vi "Main.vi"() -> ()   [LabVIEW 2020, in "ZLG_CAN.lvlib"]
doc: "This template is based off of the Queued Message Handler design pattern and the Queued Message Handler project template that ships with LabVIEW.\n\nThe main difference is that the queue is private to this module and communication between modules is performed via Broadcast and Request events.\n\nRequest events are wrapped in public API methods and are handled in the Event Handling Loop (EHL) of this VI. Any module can register for Broadcast events sent by this module. The EHL generates messages based on user interface actions.\n\nThe Message Handling Loop (MHL) processes messages generated by the EHL, or by other messages. The messages are string values, so new messages can be added easily to the Message Cases case structure in the MHL. Each message cluster can also provide an optional value for Message Data, which is a variant that can be converted to whatever message-specific data is required.\n_____\nBased on Delacor QMH Project Template 4.1.0.59."
uses:
  ZLG_CAN.lvlib
  <vilib>/Delacor/Delacor QMH/Libraries/Module Admin_class/Delacor_lib_QMH_Module Admin.lvclass
  CAN_OBJ_R.ctl
  Module Data--cluster.ctl
  <vilib>/Delacor/Delacor QMH/Libraries/Message Queue_class/Delacor_lib_QMH_Message Queue.lvclass/Delacor_lib_QMH_Message Queue.ctl
  Stop Argument--cluster.ctl
  <vilib>/Delacor/Delacor QMH/Libraries/Module Admin_class/Delacor_lib_QMH_Module Admin.lvclass/Delacor_lib_QMH_Module Admin.ctl
  Open_CAN Argument--cluster.ctl
  Init_CAN Argument--cluster.ctl
  Start_CAN Argument--cluster.ctl
  Start_CAN (Reply Payload)--cluster.ctl
  Sent_CAN Argument--cluster.ctl
  CAN_Frame.ctl
  Close_CAN Argument--cluster.ctl
  Reset_CAN Argument--cluster.ctl
  Recive_CAN Argument--cluster.ctl
  <vilib>/Utility/miscctls.llb/LVPointTypeDef.ctl
  CAN_OBJ_T.ctl
  <vilib>/Delacor/Delacor QMH/Libraries/Message Queue_class/Delacor_lib_QMH_Enqueue Message (Single).vi
  <vilib>/Delacor/Delacor QMH/Libraries/Module Admin_class/Delacor_lib_QMH_Get External Launch.vi
  <vilib>/Utility/error.llb/Error Cluster From Error Code.vi
  <vilib>/ErrorRing/Error Ring.xnode
  <vilib>/Delacor/Delacor QMH/Libraries/Message Queue_class/Delacor_lib_QMH_Message Queue.lvclass
  ControlCAN.dll
panel:
  out "CAN_OBJ_RN":T1[](array[typedef])
  out "CAN 通道":u32
  out "索引":u32
  out "设备类型":u32
  in  "Simulate MHL Error":bool
  in  "Simulate EHL Error":bool
  out "error out":errorcluster
  in  "Module Admin":refnum<class "Delacor_lib_QMH_Module Admin.lvclass">
  out "Status":string
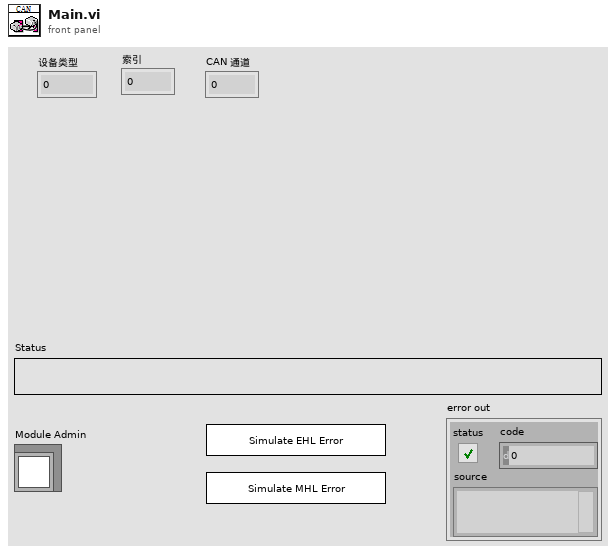
[diagram p1: front panel]
types:
  T1 = typedef "ZLG_CAN.lvlib/CAN_OBJ_R.ctl" = cluster{"ID":u32, "TimeStamp":u32, "TimeFlag":u8, "SendType":u8, "RemoteFlag":u8, "ExternFlag":u8, "DataLen":u8, "数值":u8, "数值":u8, "数值":u8, "数值":u8, "数值":u8, "数值":u8, "数值":u8, "数值":u8, "数值":u8, "数值":u8, "数值":u8}
  T2 = typedef "ZLG_CAN.lvlib/Request Events--cluster.ctl" = cluster{"Stop Module":refnum<user-event>, "Show Panel":refnum<user-event>, "Hide Panel":refnum<user-event>, "Get Module Execution Status":refnum<user-event>, "Show Diagram":refnum<user-event>, "Open_CAN":refnum<user-event>, "Init_CAN":refnum<user-event>, "Start_CAN":refnum<user-event>, "Sent_CAN":refnum<user-event>, "Close_CAN":refnum<user-event>, "Reset_CAN":refnum<user-event>, "Recive_CAN":refnum<user-event>}
  T3 = typedef "ZLG_CAN.lvlib/Module Data--cluster.ctl" = cluster{"Status":string}
  T4 = enum32{"invalid lock state", "Not Locked", "Locked (No Password)", "Password-protected"}
  T5 = typedef "ZLG_CAN.lvlib/Stop Argument--cluster.ctl" = cluster{"Origin":string, "Exit via Stop Module Req?":bool, "Wait for Module to stop?":bool}
  T6 = typedef "ZLG_CAN.lvlib/Open_CAN Argument--cluster.ctl" = cluster{"设备类型":u32, "索引":u32, "CAN 通道":u32}
  T7 = typedef "ZLG_CAN.lvlib/Init_CAN Argument--cluster.ctl" = cluster{"波特率":u32}
  T8 = typedef "ZLG_CAN.lvlib/Start_CAN Argument--cluster.ctl" = cluster{"布尔":bool, "Wait Notifier":refnum<notifier>, "wait for reply":bool}
  T9 = typedef "ZLG_CAN.lvlib/Sent_CAN Argument--cluster.ctl" = cluster{"ID":u32, "帧类型":u8, "帧格式":u8, "帧长度":u8, "CAN_FRAME":T10}
  T10 = typedef "ZLG_CAN.lvlib/CAN_Frame.ctl" = cluster{"[0]":u8, "[1]":u8, "[2]":u8, "[3]":u8, "[4]":u8, "[5]":u8, "[6]":u8, "[7]":u8}
  T11 = typedef "ZLG_CAN.lvlib/Close_CAN Argument--cluster.ctl" = cluster{"设备类型":u32, "索引":u32}
  T12 = typedef "ZLG_CAN.lvlib/Reset_CAN Argument--cluster.ctl" = cluster{"设备类型":u32, "索引":u32, "CAN 通道":u32}
  T13 = typedef "ZLG_CAN.lvlib/Recive_CAN Argument--cluster.ctl" = cluster{"布尔":bool}
  T14 = typedef "LVPointTypeDef.ctl" = cluster{"Horizontal":i16, "Vertical":i16}
  T15 = enum32{"Invalid", "Standard", "Closed", "Hidden", "Minimized", "Maximized"}
  T16 = cluster{"AccCode":u32, "AccMask":u32, "Reserved":u32, "Filter":u8, "Timing0":u8, "Timing1":u8, "Mode":u8}
  T17 = typedef "ZLG_CAN.lvlib/CAN_OBJ_T.ctl" = cluster{"ID":u32, "TimeStamp":u32, "TimeFlag":u8, "SendType":u8, "RemoteFlag":u8, "ExternFlag":u8, "DataLen":u8, "CAN_Bit_0":u8, "CAN_Bit_1":u8, "CAN_Bit_2":u8, "CAN_Bit_3":u8, "CAN_Bit_4":u8, "CAN_Bit_5":u8, "CAN_Bit_6":u8, "CAN_Bit_7":u8, "CAN_Bit_8":u8, "CAN_Bit_9":u8, "CAN_Bit_10":u8}
  T18 = typedef "ZLG_CAN.lvlib/Start_CAN (Reply Payload)--cluster.ctl" = cluster{"Success":bool, "Start_CAN_error":errorcluster}
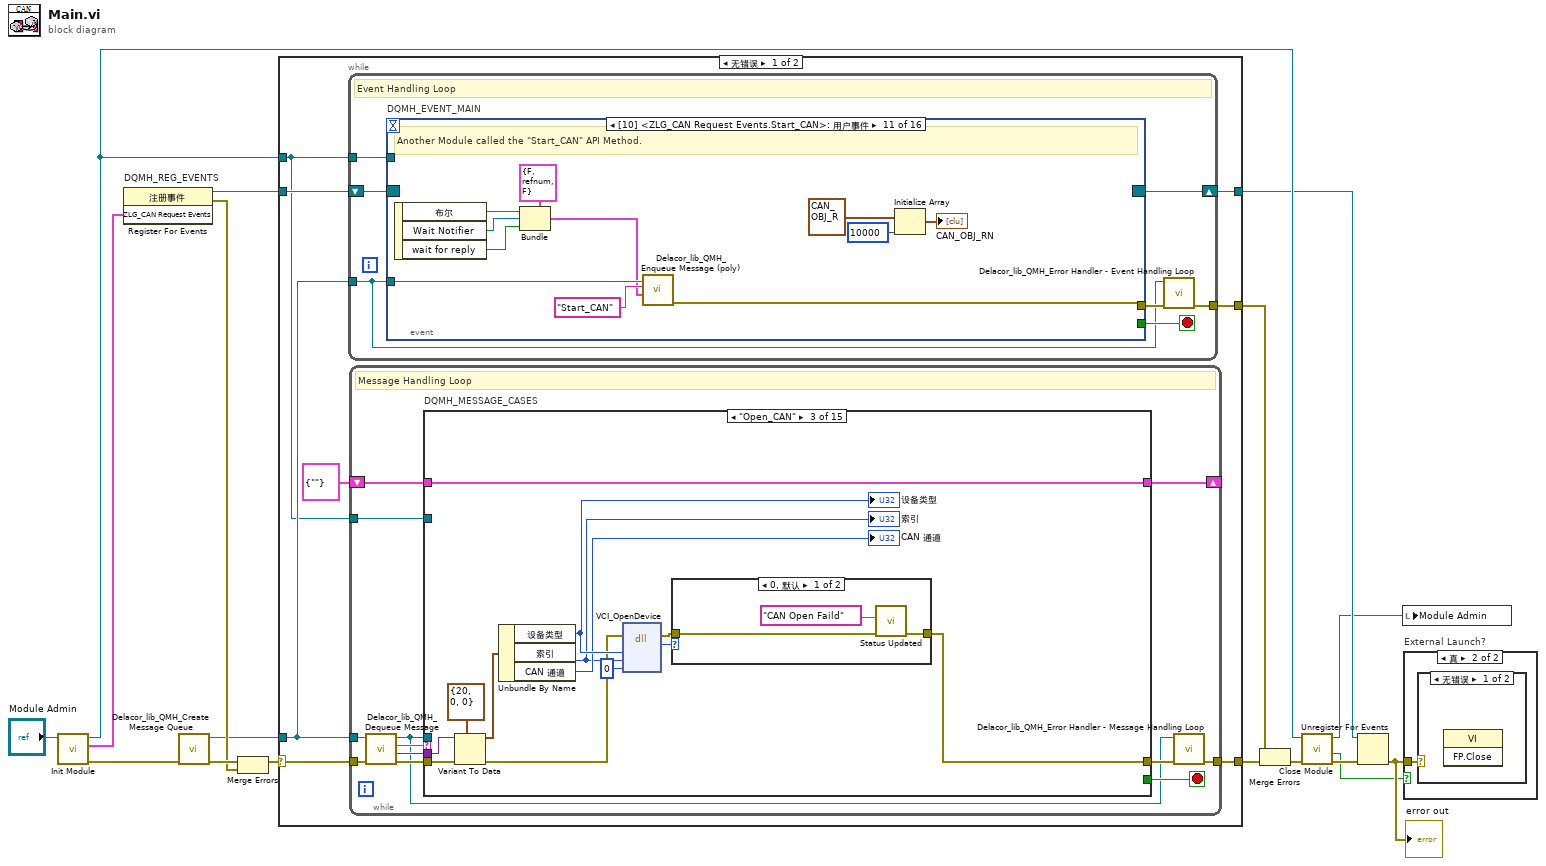
[diagram p0: block diagram]
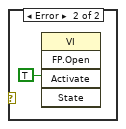
[diagram p3: hidden frame]
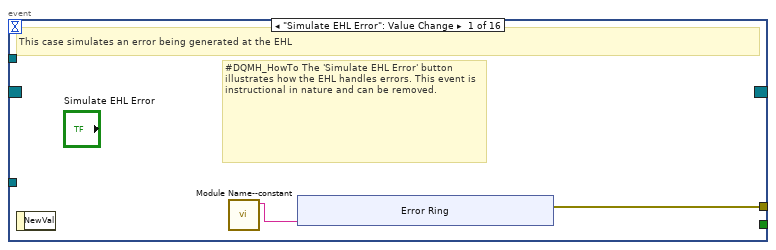
[diagram p4: hidden frame]
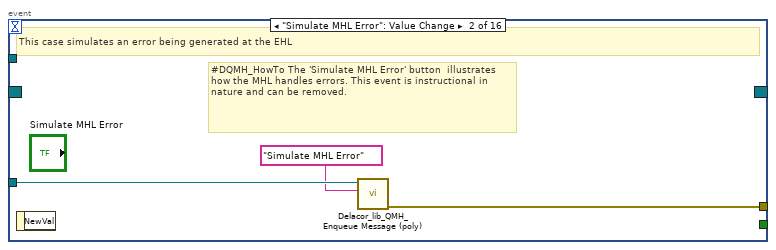
[diagram p5: hidden frame]
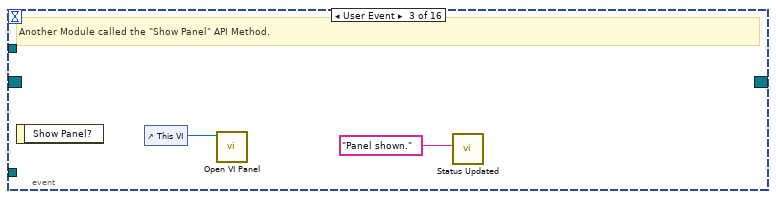
[diagram p6: hidden frame]
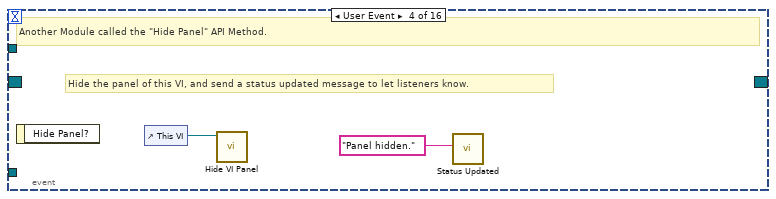
[diagram p7: hidden frame]
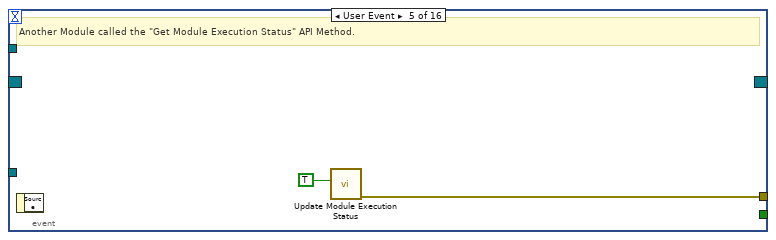
[diagram p8: hidden frame]
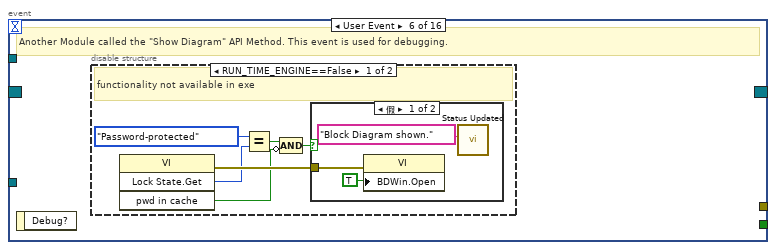
[diagram p9: hidden frame]
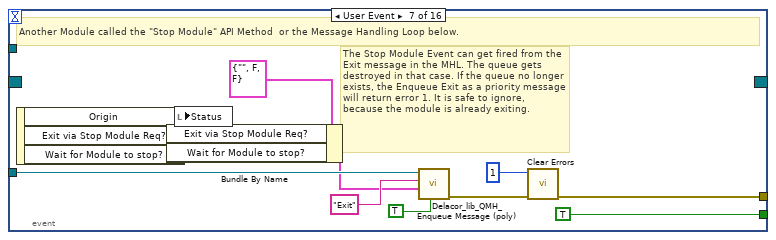
[diagram p12: hidden frame]
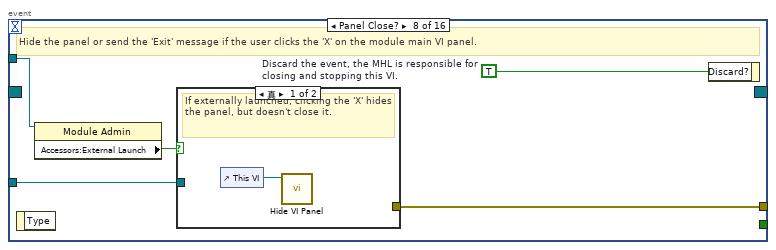
[diagram p13: hidden frame]
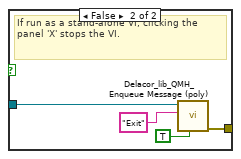
[diagram p14: hidden frame]
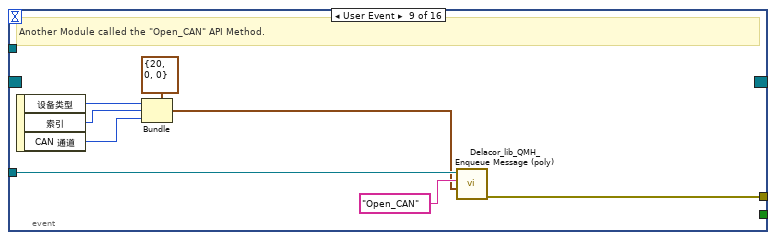
[diagram p15: hidden frame]
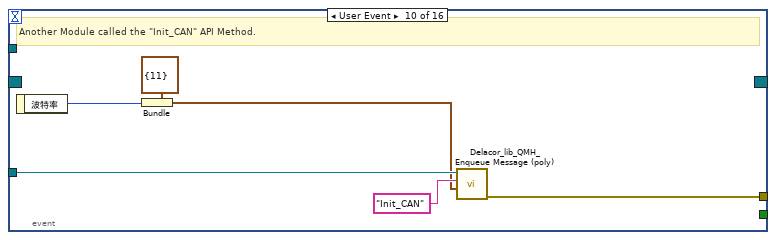
[diagram p16: hidden frame]
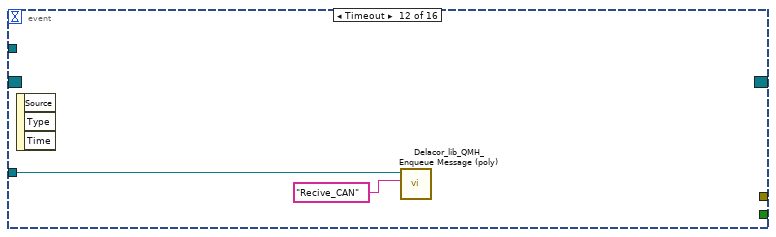
[diagram p17: hidden frame]
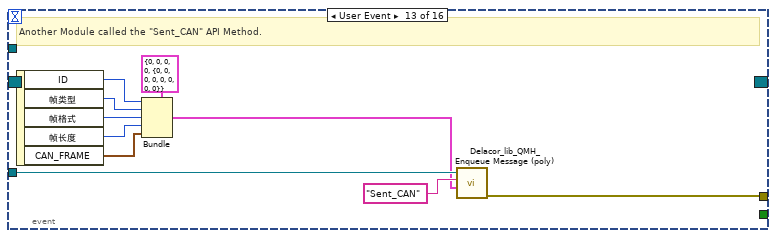
[diagram p18: hidden frame]
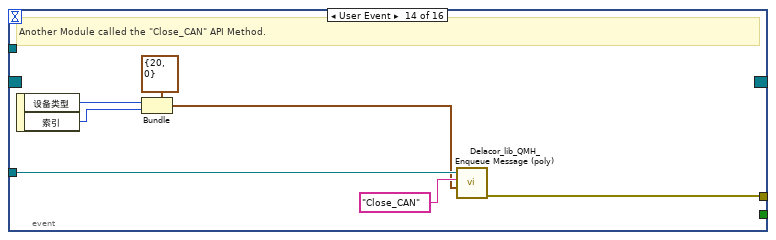
[diagram p19: hidden frame]
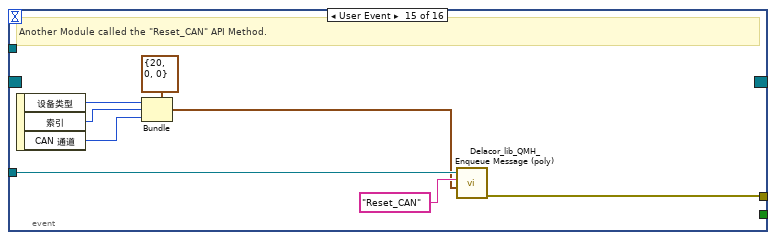
[diagram p20: hidden frame]
diagram:
  n1 = call "Init Module.vi"("Singleton Module Admin in"="Module Admin") -> ("error out"=w16:errorcluster, "ZLG_CAN Request Events"=w5:T2, "Singleton Module Admin out"=w8:refnum<class "Delacor_lib_QMH_Module Admin.lvclass">)  [unwired: 8 in]
  n2 = register-events "DQMH_REG_EVENTS"(w5) -> (reference out=w6:refnum<event-registration>, error out=w9:errorcluster)  [unwired: 2 in]
  n3 = call <vilib>:"Delacor_lib_QMH_Create Message Queue.vi"("error in"=w16) -> ("error out"=w11:errorcluster, "Message Queue"=w4:refnum<class "Delacor_lib_QMH_Message Queue.lvclass">)  [unwired: 9 in]
  n4 = Merge Errors(w11, w9) -> (w10:errorcluster)
  n5 = case shown="无错误" w10 {
    selector: w10 -> [w23 w462]
    tunnel: [w25 w462] -> w17
    tunnel: [w22 w459] -> w7
    tunnel: w6 -> [w20 w459]
    tunnel: w4 -> [w19 _]
    tunnel: [w24 _] -> w14
    tunnel: w8 -> [w18 w455]
    frame No Error {
      n6 = while {
        tunnel: w19 -> [w26]
        shift-right: [w29] -> w22
        shift-left: w20 -> [w30]
        tunnel: [w31] -> w24
        tunnel: w18 -> [w27]
        stop <- w28 stop-if-true
        # "Event Handling Loop"
        n7 = event "DQMH_EVENT_MAIN" shown="[10] <ZLG_CAN Request Events.Start_CAN>: 用户事件" {
          selector: w30 -> [_ _ _ _ _ _ _ _ _ _ _ _ _ _ _ _]
          dyn-events: [_ _ _ _ _ _ _ _ _ _ _ _ _ _ _ _] -> w29
          timeout: _ -> [_ _ _ _ _ _ _ _ _ _ _ _ _ _ _ _]
          tunnel: [_ _ _ _ _ _ TRUE ("Discard?") _ _ _ _ _ _ _ _ _] -> w28
          tunnel: w26 -> [_ w43 _ _ _ _ w67 w74 w89 w95 w106 w107 w118 w125 w133 w139]
          tunnel: [w34 w44 _ _ w50 _ w70 w76 w82 w90 w101 _ w113 w119 w128 w134] -> w32
          tunnel: w27 -> [_ _ _ _ _ _ _ w73 _ _ _ _ _ _ _ _]
          event "Simulate EHL Error": Value Change {
            # "#DQMH_HowTo The 'Simulate EHL Error' button  illustrates how the EHL handles errors. This event is instructional in nature and can be removed."
            # "This case simulates an error being generated at the EHL"
            n8 = event-data() -> ()  [unwired: 1 in, 1 out]
            n9 = call "Module Name--constant.vi"() -> ("Module Name"=w33:string)  [unwired: 11 in]
            n10 = xnode "Error Ring"("参数 0"=w33) -> ("错误输出"=w34:errorcluster)
          }
          event "Simulate MHL Error": Value Change {
            # "#DQMH_HowTo The 'Simulate MHL Error' button  illustrates how the MHL handles errors. This event is instructional in nature and can be removed."
            # "This case simulates an error being generated at the EHL"
            n11 = event-data() -> ()  [unwired: 1 in, 1 out]
            n12 = call-poly <vilib>:"Delacor_lib_QMH_Enqueue Message (poly).vi"("Message"="Simulate MHL Error", "Message Queue in"=w43) -> ("error out"=w44:errorcluster)  [unwired: 8 in, 1 out]
          }
          event User Event {
            # "Another Module called the \"Show Panel\" API Method."
            n13 = event-data() -> ()  [unwired: 1 in, 1 out]
            n14 = control-ref of="This VI"() -> (w46:refnum<vi>)
            n15 = call "Open VI Panel.vi"("VI"=w46) -> ()  [unwired: 10 in, 1 out]
            n16 = call "Status Updated.vi"("Status"="Panel shown." ("format string")) -> ()  [unwired: 10 in, 1 out]
          }
          event User Event {
            # "Hide the panel of this VI, and send a status updated message to let listeners know."
            # "Another Module called the \"Hide Panel\" API Method."
            n17 = event-data() -> ()  [unwired: 1 in, 1 out]
            n18 = control-ref of="This VI"() -> (w48:refnum<vi>)
            n19 = call "Hide VI Panel.vi"("VI"=w48) -> ()  [unwired: 10 in, 1 out]
            n20 = call "Status Updated.vi"("Status"="Panel hidden." ("format string")) -> ()  [unwired: 10 in, 1 out]
          }
          event User Event {
            # "Another Module called the \"Get Module Execution Status\" API Method."
            n21 = event-data() -> ()  [unwired: 1 in, 1 out]
            n22 = call "Update Module Execution Status.vi"("Running?"=TRUE) -> ("error out"=w50:errorcluster)  [unwired: 10 in]
          }
          event User Event {
            # "Another Module called the \"Show Diagram\" API Method. This event is used for debugging."
            n23 = event-data() -> ()  [unwired: 1 in, 1 out]
            n24 = disable-structure shown="RUN_TIME_ENGINE==False" {
              frame condition #0 (active) {
                # "functionality not available in exe"
                n25 = invoke class="VI" method="Lock State.Get"() -> (error out=w56:errorcluster, "Get Lock State"=w55:T4, "pwd in cache"=w52:bool)  [unwired: 4 in, 1 out]
                n26 = Equal?(x=T4."Password-protected", y=w55) -> (x = y?=w53:bool)
                n27 = Compound Arithmetic op=AND(w53, invert w52) -> (w51:bool)
                n28 = case "条件结构" shown="假" w51 {
                  tunnel: w56 -> [w59 _]
                  frame False {
                    n29 = property class="VI"(error in=w59, "BDWin.Open"=TRUE ("Block Diagram Window:Open")) -> ()  [unwired: 1 in, 2 out]
                    n30 = call "Status Updated.vi"("Status"="Block Diagram shown." ("format string")) -> ()  [unwired: 10 in, 1 out]
                  }
                  frame True {
                    # "Password-protected VI, and the password is not in the cache. Do not show the diagram."
                  }
                }
              }
              frame condition #1 {
              }
            }
          }
          event User Event {
            # "The Stop Module Event can get fired from the Exit message in the MHL. The queue gets destroyed in that case. If the queue no longer exists, the Enqueue Exit as a priority message will return error 1. It is safe to ignore, because the module is already exiting."
            # "Another Module called the \"Stop Module\" API Method  or the Message Handling Loop below."
            n31 = event-data() -> ("Origin"=w66:string, "Exit via Stop Module Req?"=w62:bool, "Wait for Module to stop?"=w61:bool)  [unwired: 1 in]
            n32 = Bundle By Name(cluster=T5 {"Origin"="", "Exit via Stop Module Req?"=FALSE, "Wait for Module to stop?"=FALSE} ("Stop Argument"), "Exit via Stop Module Req?"=w62, "Wait for Module to stop?"=w61) -> (w60:T5)
            n33 = local write "Status"(w66) -> ()
            n34 = call-poly <vilib>:"Delacor_lib_QMH_Enqueue Message (poly).vi"("Priority Message? (F)"=TRUE, "Message Data"=w60, "Message"="Exit", "Message Queue in"=w67) -> ("error out"=w71:errorcluster)  [unwired: 6 in, 1 out]
            n35 = call <vilib>:"Clear Errors.vi"("error in (no error)"=w71, "specific error code to clear (0: all)"=1) -> ("error out"=w70:errorcluster)  [unwired: 4 in, 1 out]
          }
          event Panel Close? {
            w75 = TRUE  # Discard the event, the MHL is responsible for closing and stopping this VI.
            # "Hide the panel or send the 'Exit' message if the user clicks the 'X' on the module main VI panel."
            n36 = event-data() -> ()  [unwired: 1 in, 1 out]
            n37 = property class="Module Admin"(reference=w73) -> ("Accessors:External Launch"=w72:bool)  [unwired: 1 in, 2 out]
            n38 = case "条件结构" shown="真" w72 {
              tunnel: w74 -> [_ w80]
              tunnel: [_ w81] -> w76
              frame True {
                # "If externally launched, clicking the 'X' hides the panel, but doesn't close it."
                n39 = control-ref of="This VI"() -> (w77:refnum<vi>)
                n40 = call "Hide VI Panel.vi"("VI"=w77) -> ()  [unwired: 10 in, 1 out]
              }
              frame False {
                # "If run as a stand-alone VI, clicking the panel 'X' stops the VI."
                n41 = call-poly <vilib>:"Delacor_lib_QMH_Enqueue Message (poly).vi"("Priority Message? (F)"=TRUE, "Message"="Exit", "Message Queue in"=w80) -> ("error out"=w81:errorcluster)  [unwired: 7 in, 1 out]
              }
            }
            n42 = event-data("Discard?"=w75) -> ()  [unwired: 1 in, 1 out]
          }
          event User Event {
            # "Another Module called the \"Open_CAN\" API Method."
            n43 = event-data() -> ("设备类型"=w85:u32, "索引"=w84:u32, "CAN 通道"=w83:u32)  [unwired: 1 in]
            n44 = Bundle(cluster=T6 {"设备类型"=20, "索引"=0, "CAN 通道"=0} ("Open_CAN Argument"), "设备类型"=w85, "索引"=w84, "CAN 通道"=w83) -> (w86:T6)
            n45 = call-poly <vilib>:"Delacor_lib_QMH_Enqueue Message (poly).vi"("Message Data"=w86, "Message"="Open_CAN", "Message Queue in"=w89) -> ("error out"=w82:errorcluster)  [unwired: 7 in, 1 out]
          }
          event User Event {
            # "Another Module called the \"Init_CAN\" API Method."
            n46 = event-data() -> ("波特率"=w91:u32)  [unwired: 1 in]
            n47 = Bundle(cluster=T7 {"波特率"=11} ("Init_CAN Argument"), "波特率"=w91) -> (w92:T7)
            n48 = call-poly <vilib>:"Delacor_lib_QMH_Enqueue Message (poly).vi"("Message Data"=w92, "Message"="Init_CAN", "Message Queue in"=w95) -> ("error out"=w90:errorcluster)  [unwired: 7 in, 1 out]
          }
          event User Event {
            # "Another Module called the \"Start_CAN\" API Method."
            n49 = event-data() -> ("布尔"=w102:bool, "Wait Notifier"=w100:refnum<notifier>, "wait for reply"=w99:bool)  [unwired: 1 in]
            n50 = Bundle(cluster=T8 {"布尔"=FALSE, "Wait Notifier"=refnum, "wait for reply"=FALSE} ("Start_CAN Argument"), "布尔"=w102, "Wait Notifier"=w100, "wait for reply"=w99) -> (w103:T8)
            n51 = call-poly <vilib>:"Delacor_lib_QMH_Enqueue Message (poly).vi"("Message Data"=w103, "Message"="Start_CAN", "Message Queue in"=w106) -> ("error out"=w101:errorcluster)  [unwired: 7 in, 1 out]
            n52 = Initialize Array(T1 {"ID"=0, "TimeStamp"=0, "TimeFlag"=0, "SendType"=1, "RemoteFlag"=0, "ExternFlag"=0, "DataLen"=8, "数值"=0, "数值"=0, "数值"=0, "数值"=0, "数值"=0, "数值"=0, "数值"=0, "数值"=0, "数值"=0, "数值"=0, "数值"=0} ("CAN_OBJ_R"), 10000 ("维数大小")) -> (→"CAN_OBJ_RN":T1[])
          }
          event Timeout {
            n53 = event-data() -> ()  [unwired: 1 in, 3 out]
            n54 = call-poly <vilib>:"Delacor_lib_QMH_Enqueue Message (poly).vi"("Message"="Recive_CAN", "Message Queue in"=w107) -> ()  [unwired: 8 in, 2 out]
          }
          event User Event {
            # "Another Module called the \"Sent_CAN\" API Method."
            n55 = event-data() -> ("ID"=w114:u32, "帧类型"=w112:u8, "帧格式"=w111:u8, "帧长度"=w110:u8, "CAN_FRAME"=w109:T10)  [unwired: 1 in]
            n56 = Bundle(cluster=T9 {"ID"=0, "帧类型"=0, "帧格式"=0, "帧长度"=0, "CAN_FRAME"={"[0]"=0, "[1]"=0, "[2]"=0, "[3]"=0, "[4]"=0, "[5]"=0, "[6]"=0, "[7]"=0}} ("Sent_CAN Argument"), "ID"=w114, "帧类型"=w112, "帧格式"=w111, "帧长度"=w110, "CAN_FRAME"=w109) -> (w115:T9)
            n57 = call-poly <vilib>:"Delacor_lib_QMH_Enqueue Message (poly).vi"("Message Data"=w115, "Message"="Sent_CAN", "Message Queue in"=w118) -> ("error out"=w113:errorcluster)  [unwired: 7 in, 1 out]
          }
          event User Event {
            # "Another Module called the \"Close_CAN\" API Method."
            n58 = event-data() -> ("设备类型"=w121:u32, "索引"=w120:u32)  [unwired: 1 in]
            n59 = Bundle(cluster=T11 {"设备类型"=20, "索引"=0} ("Close_CAN Argument"), "设备类型"=w121, "索引"=w120) -> (w122:T11)
            n60 = call-poly <vilib>:"Delacor_lib_QMH_Enqueue Message (poly).vi"("Message Data"=w122, "Message"="Close_CAN", "Message Queue in"=w125) -> ("error out"=w119:errorcluster)  [unwired: 7 in, 1 out]
          }
          event User Event {
            # "Another Module called the \"Reset_CAN\" API Method."
            n61 = event-data() -> ("设备类型"=w129:u32, "索引"=w127:u32, "CAN 通道"=w126:u32)  [unwired: 1 in]
            n62 = Bundle(cluster=T12 {"设备类型"=20, "索引"=0, "CAN 通道"=0} ("Reset_CAN Argument"), "设备类型"=w129, "索引"=w127, "CAN 通道"=w126) -> (w130:T12)
            n63 = call-poly <vilib>:"Delacor_lib_QMH_Enqueue Message (poly).vi"("Message Data"=w130, "Message"="Reset_CAN", "Message Queue in"=w133) -> ("error out"=w128:errorcluster)  [unwired: 7 in, 1 out]
          }
          event User Event {
            # "Another Module called the \"Recive_CAN\" API Method."
            n64 = event-data() -> ("布尔"=w135:bool)  [unwired: 1 in]
            n65 = Bundle(cluster=T13 {"布尔"=FALSE} ("Recive_CAN Argument"), "布尔"=w135) -> (w136:T13)
            n66 = call-poly <vilib>:"Delacor_lib_QMH_Enqueue Message (poly).vi"("Message Data"=w136, "Message"="Recive_CAN", "Message Queue in"=w139) -> ("error out"=w134:errorcluster)  [unwired: 7 in, 1 out]
          }
        }
        n67 = call-dynamic "Delacor_lib_QMH_Error Handler - Event Handling Loop.vi"("error in"=w32, "Message Queue in"=w26) -> ("dup error in"=w31:errorcluster)  [unwired: 8 in, 1 out]
      }
      n68 = while {
        tunnel: w19 -> [w142]
        shift-right: [w146] -> _
        shift-left: T3 {"Status"=""} ("Data Cluster") -> [w147]
        tunnel: w23 -> [w150]
        tunnel: [w148] -> w25
        tunnel: w18 -> [w140]
        stop <- w145 stop-if-true
        # "Message Handling Loop"
        n69 = call-dynamic "Delacor_lib_QMH_Dequeue Message.vi"("error in"=w150, "Message Queue in"=w142) -> ("error out"=w149:errorcluster, "Message Data"=w143:variant, "Message"=w144:string, "Message Queue out"=w141:refnum<class "Delacor_lib_QMH_Message Queue.lvclass">)  [unwired: 6 in]
        n70 = case "DQMH_MESSAGE_CASES" shown="\"Open_CAN\"" w144 {
          selector: w144 -> [_ _ _ _ _ _ _ _ _ _ _ _ _ _ w442]
          tunnel: w141 -> [_ _ _ _ _ _ _ _ _ _ _ _ w412 w434 _]
          tunnel: w149 -> [w169 w173 w186 w212 w284 w306 w324 w348 w366 w395 w397 w402 w419 w440 w444]
          tunnel: [w167 w173 w176 w193 w252 w298 w318 w340 w359 w394 w397 w401 w415 w437 w445] -> w151
          tunnel: w147 -> [w158 w172 w185 w211 w283 w305 w323 w347 w365 w393 w396 w399 w414 w433 w443]
          tunnel: [w157 w172 w185 w211 w283 w305 w323 w347 w365 w393 w396 w399 w414 w433 w443] -> w146
          tunnel: [_ _ _ _ _ _ _ _ _ _ _ _ _ w432 _] -> w145
          tunnel: w143 -> [_ _ w184 w210 w282 w304 w322 w346 w364 _ _ _ w413 w431 _]
          tunnel: w140 -> [w159 _ _ _ _ _ _ _ _ _ _ _ w411 w426 _]
          frame "Initialize" {
            w152 = "Initial Message" ("Initial Message")
            # "#CodeNeeded - Initialize the appearance of the front panel."
            # "#CodeNeeded - Initialize your state data here."
            # "Initialize - Any operation that needs to be done before the module can receive messages. Synchronize Caller Events.vi will inform Start Module.vi that the module has launched and is ready to receive messages. Module Did Init.vi will broadcast that the module initialized."
            n71 = call "Synchronize Caller Events.vi"("error in (no error)"=w169, "Singleton Module Admin in"=w159) -> ("error out"=w168:errorcluster, "Singleton Module Admin out"=w154:refnum<class "Delacor_lib_QMH_Module Admin.lvclass">)  [unwired: 8 in]
            n72 = property class="Module Admin"(reference=w154) -> ("Accessors:External Launch"=w163:bool)  [unwired: 1 in, 2 out]
            n73 = Select(t=T15."Hidden" ("State"), s=w163, f=T15."Standard" ("State")) -> (s? t:f=w160:T15)
            n74 = call "Module Name--constant.vi"() -> ("Module Name"=w166:string)  [unwired: 11 in]
            n75 = property class="VI"("Front Panel.Title"=w166) -> (reference out=w165:refnum<vi>, error out=w171:errorcluster)  [unwired: 2 in]
            n76 = call "Module Name--constant.vi"() -> ("Module Name"=w155:string)  [unwired: 11 in]
            n77 = invoke class="VI" method="FP.Open"(reference=w165, error in=w171, "State"=w160) -> (reference out=w164:refnum<vi>, error out=w170:errorcluster)  [unwired: 2 in, 3 out]
            n78 = Bundle By Name(cluster=w158, "Status"=w152) -> (w157:T3)
            n79 = call "Module Did Init.vi"("error in (no error)"=w168, "Initialized?"=TRUE, "Origin"=w155) -> ("error out"=w167:errorcluster)  [unwired: 8 in]
            n80 = invoke class="VI" method="FP.Center"(reference=w164, error in=w170) -> ()  [unwired: 1 in, 3 out]
            n81 = property on="Pane" class="Pane"("Origin"=T14 {"Horizontal"=0, "Vertical"=0}) -> ()  [unwired: 2 in, 2 out]
            "Status" <- w152
          }
          frame "--- Module Specific ---" {
            # "Separator -- The following cases handle messages specific to this Module."
          }
          frame "Open_CAN" {
            n82 = Variant To Data(error in=w186, type=T6 {"设备类型"=20, "索引"=0, "CAN 通道"=0} ("Open_CAN Argument"), Variant=w184) -> (data=w182:T6, error out=w179:errorcluster)
            n83 = Unbundle By Name(w182) -> ("设备类型"=w181:u32, "索引"=w174:u32, "CAN 通道"=→"CAN 通道":u32)
            "设备类型" <- w181
            "索引" <- w174
            n84 = dll-call lib="PTH2rabs CUsers\n终极BOSS\tDocumentsCEPSLV180648-11中间轴装配SourcesOtherZLG_CANControlCAN.dll" fn="VCI_OpenDevice"(error in=w179, "DevType"=w181, "DevIndex"=w174, "Reserved"=u32 0) -> (error out=w177:errorcluster, "返回类型"=w178:u32)  [unwired: 5 in, 1 out]
            n85 = case shown="0, 默认" w178 {
              tunnel: w177 -> [w188 w191]
              tunnel: [w187 w190] -> w176
              frame 0, Default {
                n86 = call "Status Updated.vi"("error in (no error)"=w188, "Status"="CAN Open Faild" ("format string")) -> ("error out"=w187:errorcluster)  [unwired: 9 in]
              }
              frame 1 {
                n87 = call "Status Updated.vi"("error in (no error)"=w191, "Status"="CAN Open Success" ("format string")) -> ("error out"=w190:errorcluster)  [unwired: 9 in]
              }
            }
          }
          frame "Init_CAN" {
            w202 = u32 0 ("Reserved")
            n88 = Variant To Data(error in=w212, type=T7 {"波特率"=11} ("Init_CAN Argument"), Variant=w210) -> (data=w208:T7, error out=w196:errorcluster)
            n89 = Unbundle By Name(w208) -> ("波特率"=w201:u32)
            n90 = case shown="4" w201 {
              tunnel: [u8 191 ("BTR0") 49 24 135 9 131 4 3 250 1 128 0 128 0 0 1] -> w207
              tunnel: [u8 255 ("BTR1") 28 28 255 28 255 28 28 129 28 250 28 182 22 20 1] -> w206
              frame 0 {
              }
              frame 1 {
              }
              frame 2 {
              }
              frame 3 {
              }
              frame 4 {
              }
              frame 5 {
              }
              frame 6 {
              }
              frame 7 {
              }
              frame 8 {
              }
              frame 9 {
              }
              frame 10 {
              }
              frame 11 {
              }
              frame 12 {
              }
              frame 13 {
              }
              frame 14 {
              }
              frame 15, Default {
              }
            }
            n91 = local read "设备类型"() -> (w197:u32)
            n92 = local read "索引"() -> (w198:u32)
            n93 = local read "CAN 通道"() -> (w199:u32)
            n94 = Bundle(cluster=T16 {"AccCode"=0, "AccMask"=4294967295, "Reserved"=0, "Filter"=0, "Timing0"=3, "Timing1"=28, "Mode"=0} ("VCI_INIT_CONFIG"), "AccCode"=u32 0 ("验收码"), "AccMask"=u32 4294967295 ("屏蔽码"), "Reserved"=w202, "Filter"=w202, "Timing0"=w207, "Timing1"=w206, "Mode"=w202) -> (w200:T16)
            n95 = dll-call lib="PTH2rabs CUsers\n终极BOSS\tDocumentsCEPSLV180648-11中间轴装配SourcesOtherZLG_CANControlCAN.dll" fn="VCI_InitCAN"(error in=w196, "DeviceType"=w197, "DeviceInd"=w198, "CANInd"=w199, "pInitConfig"=w200) -> (error out=w194:errorcluster, "返回类型"=w195:u32)  [unwired: 6 in, 1 out]
            n96 = case shown="1" w195 {
              tunnel: w194 -> [w214 w217]
              tunnel: [w213 w216] -> w193
              frame 0, Default {
                n97 = call "Status Updated.vi"("error in (no error)"=w214, "Status"="CAN Init Faild" ("format string")) -> ("error out"=w213:errorcluster)  [unwired: 9 in]
              }
              frame 1 {
                n98 = call "Status Updated.vi"("error in (no error)"=w217, "Status"="CAN Init Success" ("format string")) -> ("error out"=w216:errorcluster)  [unwired: 9 in]
              }
            }
          }
          frame "Sent_CAN" {
            w271 = u8 0 ("CAN_Bit_7")
            w274 = u8 0 items=["正常发送", "单次发送", "自发自收", "单次自发自收"] ("发送类型")
            n99 = Variant To Data(error in=w284, type=T9 {"ID"=0, "帧类型"=0, "帧格式"=0, "帧长度"=0, "CAN_FRAME"={"[0]"=0, "[1]"=0, "[2]"=0, "[3]"=0, "[4]"=0, "[5]"=0, "[6]"=0, "[7]"=0}} ("Sent_CAN Argument"), Variant=w282) -> (data=w280:T9, error out=w256:errorcluster)
            n100 = Unbundle By Name(w280) -> ("ID"=w278:u32, "帧类型"=w273:u8, "帧格式"=w272:u8, "帧长度"=w268:u8, "CAN_FRAME"=w269:T10)
            n101 = To Unsigned Byte Integer(number=u32 0) -> (unsigned 8bit integer=w275:u8)
            n102 = Unbundle(w269) -> ("[0]"=w267:u8, "[1]"=w266:u8, "[2]"=w265:u8, "[3]"=w264:u8, "[4]"=w263:u8, "[5]"=w262:u8, "[6]"=w261:u8, "[7]"=w260:u8)
            n103 = Bundle(cluster=T17 {"ID"=0, "TimeStamp"=0, "TimeFlag"=0, "SendType"=0, "RemoteFlag"=0, "ExternFlag"=0, "DataLen"=0, "CAN_Bit_0"=0, "CAN_Bit_1"=0, "CAN_Bit_2"=0, "CAN_Bit_3"=0, "CAN_Bit_4"=0, "CAN_Bit_5"=0, "CAN_Bit_6"=0, "CAN_Bit_7"=0, "CAN_Bit_8"=0, "CAN_Bit_9"=0, "CAN_Bit_10"=0} ("VCI_CAN_OBJ_T"), "ID"=w278, "TimeStamp"=u32 0, "TimeFlag"=w275, "SendType"=w274, "RemoteFlag"=w273, "ExternFlag"=w272, "DataLen"=w268, "CAN_Bit_0"=w267, "CAN_Bit_1"=w266, "CAN_Bit_2"=w265, "CAN_Bit_3"=w264, "CAN_Bit_4"=w263, "CAN_Bit_5"=w262, "CAN_Bit_6"=w261, "CAN_Bit_7"=w260, "CAN_Bit_8"=w271, "CAN_Bit_9"=w271, "CAN_Bit_10"=w271) -> (w270:T17)
            n104 = local read "设备类型"() -> (w257:u32)
            n105 = local read "索引"() -> (w259:u32)
            n106 = local read "CAN 通道"() -> (w258:u32)
            n107 = dll-call lib="PTH2rabs CUsers\n终极BOSS\tDocumentsCEPSLV180648-11中间轴装配SourcesOtherZLG_CANControlCAN.dll" fn="VCI_Transmit"(error in=w256, "DeviceType"=w257, "DeviceInd"=w259, "CANInd"=w258, "pSend"=w270, "Len"=u32 1) -> (error out=w253:errorcluster, "return type"=w254:u32, "pSend"=w251:T17)  [unwired: 6 in, 1 out]
            n108 = case shown="1" w254 {
              tunnel: w253 -> [w286 w294]
              tunnel: [w285 w292] -> w252
              tunnel: w251 -> [_ w290]
              frame 0, Default {
                n109 = call "Status Updated.vi"("error in (no error)"=w286, "Status"="CAN Sent Success" ("format string")) -> ("error out"=w285:errorcluster)  [unwired: 9 in]
              }
              frame 1 {
                n110 = call "Status Updated.vi"("error in (no error)"=w294, "Status"="CAN Sent Success" ("format string")) -> ("error out"=w293:errorcluster)  [unwired: 9 in]
                n111 = Build Array(w290) -> (w289:T17[])
                n112 = call "CAN_Recive.vi"("error in (no error)"=w293, "T?R"=TRUE, "CAN_OBJ_RN"=w289, "NUM"=u16 1) -> ("error out"=w292:errorcluster)  [unwired: 7 in]
              }
            }
          }
          frame "Close_CAN" {
            n113 = Variant To Data(error in=w306, type=T11 {"设备类型"=20, "索引"=0} ("Close_CAN Argument"), Variant=w304) -> (data=w302:T11, error out=w299:errorcluster)
            n114 = Unbundle By Name(w302) -> ("设备类型"=w301:u32)
            n115 = dll-call lib="PTH2rabs CUsers\n终极BOSS\tDocumentsCEPSLV180648-11中间轴装配SourcesOtherZLG_CANControlCAN.dll" fn="VCI_CloseDevice"(error in=w299, "DeviceType"=w301, "DeviceInd"=u32 0) -> (error out=w300:errorcluster, "返回类型"=w297:u32)  [unwired: 4 in, 1 out]
            n116 = case shown="1" w297 {
              tunnel: w300 -> [w308 w311]
              tunnel: [w307 w310] -> w298
              frame 0, Default {
                n117 = call "Status Updated.vi"("error in (no error)"=w308, "Status"="CAN Close Faild" ("format string")) -> ("error out"=w307:errorcluster)  [unwired: 9 in]
              }
              frame 1 {
                n118 = call "Status Updated.vi"("error in (no error)"=w311, "Status"="CAN Close Success" ("format string")) -> ("error out"=w310:errorcluster)  [unwired: 9 in]
              }
            }
          }
          frame "Reset_CAN" {
            n119 = Variant To Data(error in=w324, type=T12 {"设备类型"=20, "索引"=0, "CAN 通道"=0} ("Reset_CAN Argument"), Variant=w322) -> (data=w320:T12, error out=w319:errorcluster)
            n120 = Unbundle By Name(w320) -> ("设备类型"=w315:u32, "索引"=w314:u32, "CAN 通道"=w313:u32)
            n121 = dll-call lib="PTH2rabs CUsers\n终极BOSS\tDocumentsCEPSLV180648-11中间轴装配SourcesOtherZLG_CANControlCAN.dll" fn="VCI_ResetCAN"(error in=w319, "DeviceType"=w315, "DeviceInd"=w314, "CANInd"=w313) -> (error out=w316:errorcluster, "返回类型"=w317:u32)  [unwired: 5 in, 1 out]
            n122 = case shown="1" w317 {
              tunnel: w316 -> [w325 w329]
              tunnel: [w326 w328] -> w318
              frame 0, Default {
                n123 = call "Status Updated.vi"("error in (no error)"=w325, "Status"="CAN Reset Faild" ("format string")) -> ("error out"=w326:errorcluster)  [unwired: 9 in]
              }
              frame 1 {
                n124 = call "Status Updated.vi"("error in (no error)"=w329, "Status"="CAN Reset Success" ("format string")) -> ("error out"=w328:errorcluster)  [unwired: 9 in]
              }
            }
          }
          frame "Start_CAN" {
            n125 = Variant To Data(error in=w348, type=T8 {"布尔"=FALSE, "Wait Notifier"=refnum, "wait for reply"=FALSE} ("Start_CAN Argument"), Variant=w346) -> (data=w344:T8, error out=w334:errorcluster)
            n126 = Unbundle By Name(w344) -> ("Wait Notifier"=w343:refnum<notifier>, "wait for reply"=w333:bool)
            n127 = local read "CAN 通道"() -> (w338:u32)
            n128 = local read "设备类型"() -> (w339:u32)
            n129 = local read "索引"() -> (w335:u32)
            n130 = dll-call lib="PTH2rabs CUsers\n终极BOSS\tDocumentsCEPSLV180648-11中间轴装配SourcesOtherZLG_CANControlCAN.dll" fn="VCI_StartCAN"(error in=w334, "DeviceType"=w339, "DeviceInd"=w335, "CANInd"=w338) -> (error out=w337:errorcluster, "返回类型"=w336:u32)  [unwired: 5 in, 1 out]
            n131 = case shown="1" w336 {
              tunnel: w337 -> [w351 w355]
              tunnel: [w350 w354] -> w331
              tunnel: [FALSE TRUE] -> w332
              frame 0, Default {
                n132 = call "Status Updated.vi"("error in (no error)"=w351, "Status"="CAN Start Faild" ("format string")) -> ("error out"=w350:errorcluster)  [unwired: 9 in]
              }
              frame 1 {
                n133 = call "Status Updated.vi"("error in (no error)"=w355, "Status"="CAN Start Success" ("format string")) -> ("error out"=w354:errorcluster)  [unwired: 9 in]
              }
            }
            n134 = Bundle By Name(cluster=T18 {"Success"=FALSE, "Start_CAN_error"={"status"=FALSE, "code"=0, "source"=""}} ("Start_CAN (Reply Payload)"), "Success"=w332, "Start_CAN_error"=w331) -> (w342:T18)
            n135 = case shown="真" w333 {
              tunnel: w343 -> [_ w358]
              tunnel: w342 -> [_ w357]
              frame False {
              }
              frame True {
                n136 = Send Notification(notification=w357, notifier=w358) -> ()  [unwired: 1 in, 2 out]
              }
            }
            n137 = Merge Errors(w334, w331) -> (w340:errorcluster)
          }
          frame "Recive_CAN" {
            n138 = Variant To Data(error in=w366, type=T13 {"布尔"=FALSE} ("Recive_CAN Argument"), Variant=w364) -> (data=w362:T13, error out=w360:errorcluster)
            n139 = Unbundle By Name(w362) -> ("布尔"=w361:bool)
            n140 = case shown="真" w361 {
              tunnel: w360 -> [w367 w369]
              tunnel: [w367 w368] -> w359
              frame False {
              }
              frame True {
                n141 = local read "CAN 通道"() -> (w372:u32)
                n142 = local read "设备类型"() -> (w374:u32)
                n143 = local read "索引"() -> (w373:u32)
                n144 = dll-call lib="PTH2rabs CUsers\n终极BOSS\tDocumentsCEPSLV180648-11中间轴装配SourcesOtherZLG_CANControlCAN.dll" fn="VCI_GetReceiveNum"(error in=w369, "DeviceType"=w374, "DeviceInd"=w373, "CANInd"=w372) -> (error out=w371:errorcluster, "return type"=w370:u32)  [unwired: 5 in, 1 out]
                n145 = case shown="1, 默认" w370 {
                  selector: w370 -> [_ w376]
                  tunnel: w371 -> [w375 w379]
                  tunnel: w374 -> [_ w386]
                  tunnel: w373 -> [_ w385]
                  tunnel: w372 -> [_ w384]
                  tunnel: [w375 w377] -> w368
                  frame 0 {
                  }
                  frame 1, Default {
                    n146 = local read "CAN_OBJ_RN"() -> (w383:T1[])
                    n147 = dll-call lib="PTH2rabs CUsers\n终极BOSS\tDocumentsCEPSLV180648-11中间轴装配SourcesOtherZLG_CANControlCAN.dll" fn="VCI_Receive"(error in=w379, "DeviceType"=w386, "DeviceInd"=w385, "CANInd"=w384, "pReceive"=w383, "Len"=w376, "WaitTime"=100) -> (error out=w378:errorcluster, "return type"=w381:u32, "pReceive"=w380:T1[])  [unwired: 7 in, 1 out]
                    n148 = case shown="1" w381 {
                      tunnel: w380 -> [_ w390]
                      tunnel: w378 -> [w387 w392]
                      tunnel: [w387 w391] -> w377
                      tunnel: w376 -> [_ w389]
                      frame 0, Default {
                      }
                      frame 1 {
                        n149 = call "CAN_Recive.vi"("error in (no error)"=w392, "T?R"=FALSE, "CAN_OBJ_RN"=w390, "NUM"=w389) -> ("error out"=w391:errorcluster)  [unwired: 7 in]
                      }
                    }
                  }
                }
              }
            }
          }
          frame "---Copy This Frame---" {
            # "Duplicate this frame when creating new messages.  Change this comment in the duplicated frame to describe this message."
            n150 = Merge Errors(w395) -> (w394:errorcluster)
          }
          frame "--- Exit and Error Handling---" {
            # "Separator - The following cases handle errors and exit messages."
          }
          frame "Simulate MHL Error" {
            # "Simulate an error occurring at the MHL"
            n151 = call "Module Name--constant.vi"() -> ("Module Name"=w398:string)  [unwired: 11 in]
            n152 = xnode "Error Ring"("参数 0"=w398) -> ("错误输出"=w400:errorcluster)
            n153 = Merge Errors(w402, w400) -> (w401:errorcluster)
          }
          frame "Error" {
            # "Error - Check the error message data and respond accordingly. This message is sent by the \"Error Handler\" VIs at the end of each loop in this application."
            n154 = property class="Module Admin"(reference=w411) -> ("Accessors:External Launch"=w410:bool)  [unwired: 1 in, 2 out]
            n155 = Variant To Data(error in=w419, type=errorcluster {"status"=FALSE, "code"=0, "source"=""} ("error constant"), Variant=w413) -> (data=w420:errorcluster, error out=w417:errorcluster)
            n156 = call "Error Reported.vi"("Error"=w420) -> ()  [unwired: 10 in, 1 out]
            n157 = case shown="假" w410 {
              tunnel: [w425 _] -> w416
              tunnel: w412 -> [w423 _]
              tunnel: w420 -> [w424 _]
              frame False {
                n158 = call <vilib>:"Simple Error Handler.vi"("error in (no error)"=w424) -> ()  [unwired: 4 in, 5 out]
                n159 = call-poly <vilib>:"Delacor_lib_QMH_Enqueue Message (poly).vi"("Priority Message? (F)"=TRUE, "Message"="Exit", "Message Queue in"=w423) -> ("error out"=w425:errorcluster)  [unwired: 7 in, 1 out]
              }
              frame True {
                # "If the module was launched externally, calling the Error Reported broadcast VI is the only action performed by the \"Error\" message. The module's caller can then process the error appropriately."
              }
            }
            n160 = Merge Errors(w417, w416) -> (w415:errorcluster)
            n161 = local write "error out"(w415) -> ()
          }
          frame "Exit" {
            w430 = 91  # 91: not all Exit messages will have an argument
            w432 = TRUE  # Stop the VI
            # "Exit - Exit the application."
            n162 = Variant To Data(error in=w440, type=T5 {"Origin"="", "Exit via Stop Module Req?"=FALSE, "Wait for Module to stop?"=FALSE} ("Stop Argument"), Variant=w431) -> (data=w428:T5, error out=w436:errorcluster)
            n163 = call <vilib>:"Clear Errors.vi"("error in (no error)"=w436, "specific error code to clear (0: all)"=w430) -> ("error out"=w439:errorcluster)  [unwired: 4 in, 1 out]
            n164 = control-ref of="This VI"() -> (w427:refnum<vi>)
            n165 = call-dynamic "Delacor_lib_QMH_Release Message Queue.vi"("error in"=w439, "Message Queue"=w434) -> ("error out"=w438:errorcluster)  [unwired: 9 in]
            n166 = call "Handle Exit.vi"("Stop Argument"=w428, "Admin in"=w426, "VI reference"=w427) -> ("error out"=w435:errorcluster)  [unwired: 7 in, 1 out]
            n167 = Merge Errors(w438, w435) -> (w437:errorcluster)
          }
          frame Default {
            # "'Default' case only runs if there is a message that isn't defined in any of the other cases.  Output a programming error."
            n168 = call "Module Name--constant.vi"() -> ("Module Name"=w441:string)  [unwired: 11 in]
            n169 = xnode "Error Ring"("参数 0"=w442, "参数 1"=w441) -> ("错误输出"=w446:errorcluster)
            n170 = Merge Errors(w444, w446) -> (w445:errorcluster)
          }
        }
        n171 = call-dynamic "Delacor_lib_QMH_Error Handler - Message Handling Loop.vi"("error in"=w151, "Message Queue in"=w141) -> ("dup error in"=w148:errorcluster)  [unwired: 8 in, 1 out]
      }
    }
    frame Error {
      # "Synchronize Caller Events.vi will inform Start Module.vi that the module has launched and will let the code calling Start Module.vi register for broadcasts and would permit the caller receive the broadcast that an error occurred at launch time."
      n172 = call "Synchronize Caller Events.vi"("Singleton Module Admin in"=w455) -> ("error out"=w460:errorcluster)  [unwired: 9 in, 1 out]
      n173 = call "Module Name--constant.vi"() -> ("Module Name"=w458:string)  [unwired: 11 in]
      n174 = Format Into String(format string="An error occurred during initialization. %s is no longer running.", w458) -> (resulting string=w456:string)  [unwired: 2 in, 1 out]
      n175 = Merge Errors(w462, w460) -> (w461:errorcluster)
      n176 = call "Error Reported.vi"("Additional Information"=w456, "Error"=w461) -> ()  [unwired: 9 in, 1 out]
    }
  }
  n177 = Merge Errors(w14, w17) -> (w13:errorcluster)
  n178 = call "Close Module.vi"("error in (no error)"=w13, "Module Admin in"=w8) -> ("error out"=w15:errorcluster, "External Launch"=w1:bool, "Module Admin out"=w2:refnum<class "Delacor_lib_QMH_Module Admin.lvclass">)  [unwired: 7 in]
  n179 = Unregister For Events(event registration refnum=w7, error in=w15) -> (error out=w12:errorcluster)
  "error out" <- w12
  n180 = local write "Module Admin"(w2) -> ()
  n181 = case "External Launch?" shown="真" w1 {
    tunnel: w12 -> [_ w463]
    frame False {
    }
    frame True {
      n182 = case "条件结构" shown="无错误" w463 {
        frame No Error {
          n183 = invoke class="VI" method="FP.Close"() -> ()  [unwired: 3 in, 3 out]
        }
        frame Error {
          n184 = invoke class="VI" method="FP.Open"("Activate"=TRUE ("Activate?")) -> ()  [unwired: 4 in, 5 out]
        }
      }
    }
  }
